vi "Get Z-planes.vi"() -> (0 "Pockels vs. Z (Laser power %)":dbl[](array[numeric]) format="%#_12f", 1 "Z Planes(um)":dbl[](array[numeric]) format="%#_12f", 2 "Motor Z Planes(um)":dbl[](array[numeric]) format="%#_12f", 3 "# of Z-planes":i32, 5 "ZStack":cluster{"Zstart":dbl, "Zstop":dbl, "Zstep":dbl})   [LabVIEW 2020]
uses:
  Typedefs/Read Write Enum.ctl
panel:
  out "VI Exec time":u32
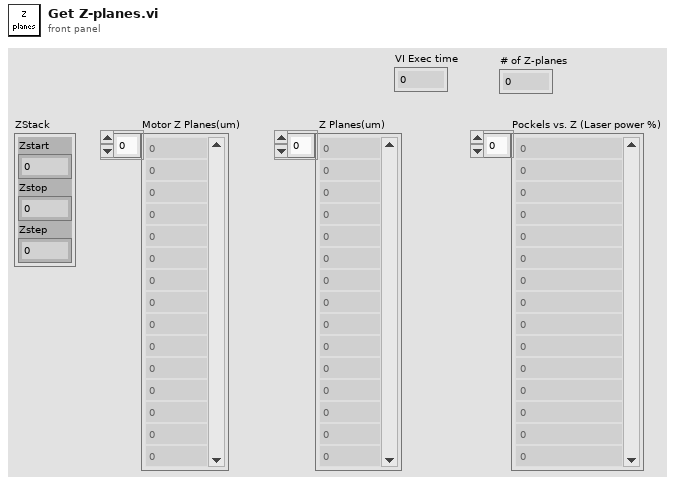
[diagram p1: front panel]
types:
  T1 = typedef "Read Write Enum.ctl" = enum16{"Read", "Write"}
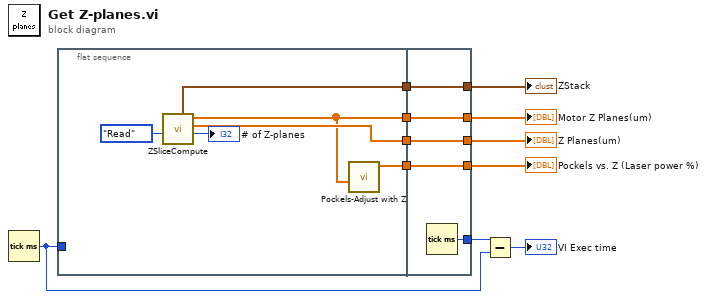
[diagram p0: block diagram]
diagram:
  n1 = Tick Count (ms)() -> (millisecond timer value=w10:u32)
  n2 = flat-sequence {
    tunnel: w10 -> [_]
    tunnel: [w16] -> w8
    tunnel: [w15] -> w5
    tunnel: [w14] -> w3
    tunnel: [w12] -> w2
    tunnel: [w22] -> w11
    tunnel: [w21] -> w7
    tunnel: w8 -> [w21]
    tunnel: [w20] -> w6
    tunnel: w5 -> [w20]
    tunnel: [w19] -> w4
    tunnel: w3 -> [w19]
    tunnel: w2 -> [w18]
    tunnel: [w18] -> w1
    frame #0 {
      n3 = call "ZSliceCompute.vi"("Function"=Read_Write_Enum."Read") -> ("# of Z-planes"=→"# of Z-planes":i32, "AOL Z Planes(um)"=w15:dbl[], "Motor Z Planes(um)"=w14:dbl[], "ZStack (um)"=w12:cluster{"Zstart":dbl, "Zstop":dbl, "Zstep":dbl})  [unwired: 7 in]
      n4 = call "Pockels-Adjust with Z.vi"("Motor Z Planes(um)"=w14) -> ("Laser power % corrected for depth"=w16:dbl[])  [unwired: 9 in, 1 out]
    }
    frame #1 {
      n5 = Tick Count (ms)() -> (millisecond timer value=w22:u32)
    }
  }
  n6 = Subtract(x=w11, y=w10) -> (x-y=→"VI Exec time":u32)
  "Pockels vs. Z (Laser power %)" <- w7
  "Motor Z Planes(um)" <- w4
  "Z Planes(um)" <- w6
  "ZStack" <- w1
